vi "Read Config.vi"(10 "Config Path":path) -> (0 "Test Table":string[][](array[string]), 1 "C_Tol":dbl, 2 "P_Tol":dbl, 3 "PSID":dbl, 5 "Excel  Template":path)   [LabVIEW 2018]
uses:
  <vilib>/Utility/config.llb/Read Key (Double).vi
  <vilib>/Utility/config.llb/Read Key (Path).vi
  <vilib>/Utility/config.llb/Read Key (String).vi
  <vilib>/Utility/config.llb/NI_LVConfig.lvlib
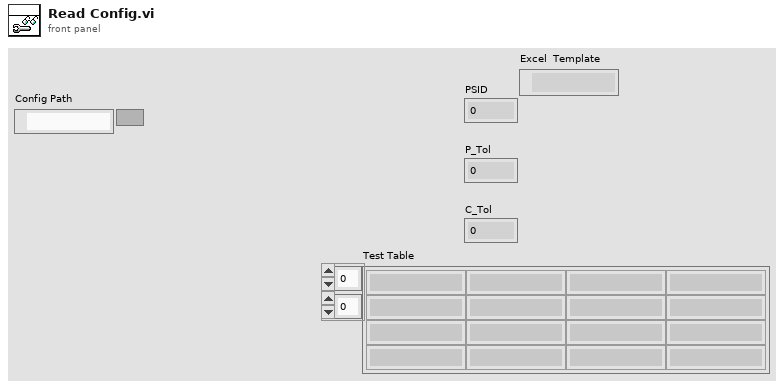
[diagram p1: front panel]
types:
  T1 = typedef "NI_LVConfig.lvlib/Config Data RefNum.ctl" = refnum<k1>
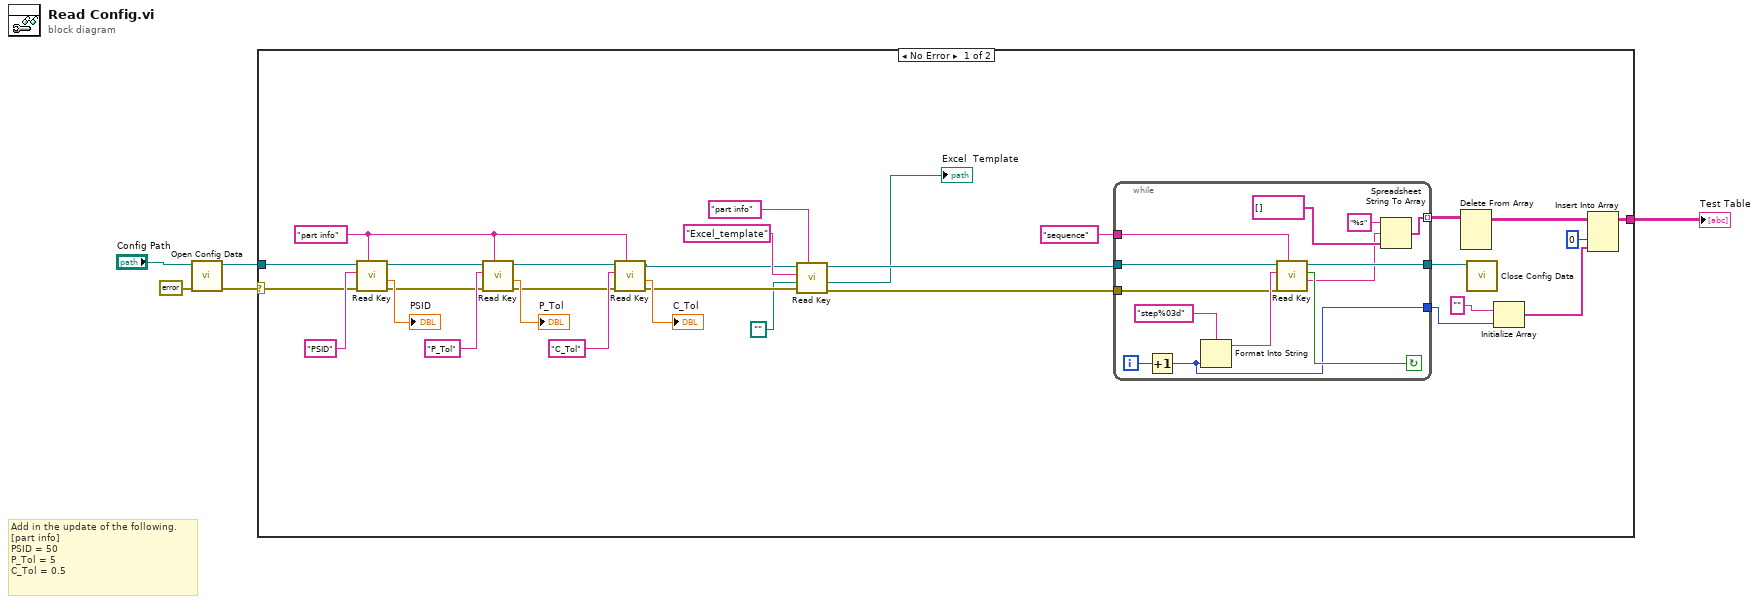
[diagram p0: block diagram]
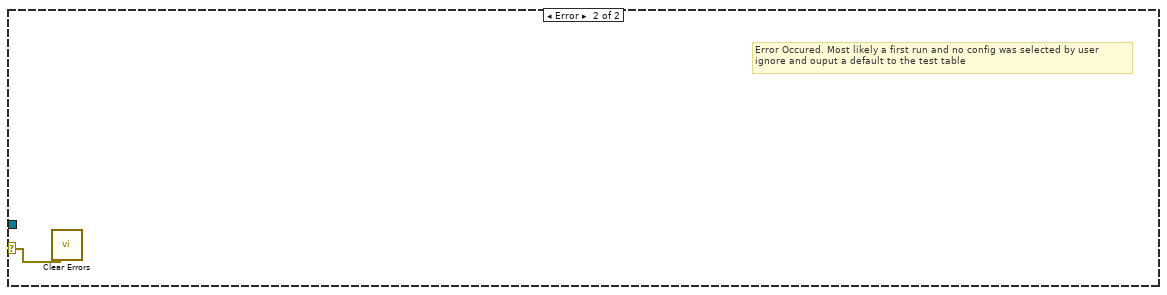
[diagram p2: hidden frame]
diagram:
  # "Add in the update of the following.\n[part info]\nPSID = 50\nP_Tol = 5\nC_Tol = 0.5"
  n1 = call <vilib>:"Open Config Data.vi"("error in (no error)"=errorcluster {"status"=FALSE, "code"=0, "source"=""}, "configuration file path"="Config Path") -> ("error out"=w2:errorcluster, "refnum"=w5:T1)  [unwired: 7 in, 1 out]
  n2 = case shown="No Error" w2 {
    selector: w2 -> [w13 w49]
    tunnel: w5 -> [w35 _]
    tunnel: [w21 _] -> w4
    frame No Error {
      w34 = "part info" ("section")
      n3 = call-poly <vilib>:"Read Key.vi"("section"=w34, "error in (no error)"=w13, "key"="PSID", "refnum"=w35) -> ("error out"=w12:errorcluster, "value"=→"PSID":dbl, "refnum out"=w27:T1)  [unwired: 4 in, 1 out]
      n4 = call-poly <vilib>:"Read Key.vi"("section"=w34, "error in (no error)"=w12, "key"="P_Tol", "refnum"=w27) -> ("error out"=w11:errorcluster, "value"=→"P_Tol":dbl, "refnum out"=w26:T1)  [unwired: 4 in, 1 out]
      n5 = call-poly <vilib>:"Read Key.vi"("section"=w34, "error in (no error)"=w11, "key"="C_Tol", "refnum"=w26) -> ("error out"=w10:errorcluster, "value"=→"C_Tol":dbl, "refnum out"=w14:T1)  [unwired: 4 in, 1 out]
      n6 = call-poly <vilib>:"Read Key.vi"("section"="part info", "error in (no error)"=w10, "default value"=path "", "key"="Excel_template", "refnum"=w14) -> ("error out"=w9:errorcluster, "value"=→"Excel  Template":path, "refnum out"=w8:T1)  [unwired: 3 in, 1 out]
      n7 = while {
        tunnel: w8 -> [w48]
        tunnel: "sequence" ("section") -> [w47]
        tunnel: [w42] -> w24
        tunnel: [w39] -> w23 mode=indexing
        tunnel: [w37] -> w20
        tunnel: w9 -> [w36]
        i -> [w46]
        stop <- w43 continue-if-true
        n8 = Increment(x=w46) -> (x+1=w37:i32)
        n9 = Format Into String(format string="step%03d", w37) -> (resulting string=w44:string)  [unwired: 2 in, 1 out]
        n10 = call-poly <vilib>:"Read Key.vi"("section"=w47, "error in (no error)"=w36, "key"=w44, "refnum"=w48) -> ("value"=w40:string, "found?"=w43:bool, "refnum out"=w42:T1)  [unwired: 4 in, 1 out]
        n11 = Spreadsheet String To Array(format string="%s", spreadsheet string=w40, array type (2D Dbl)=string[] []) -> (array=w39:string[])  [unwired: 1 in]
      }
      n12 = Delete From Array(array=w23) -> (array with subset deleted=w22:string[][])  [unwired: 3 in, 1 out]
      n13 = call <vilib>:"Close Config Data.vi"("refnum"=w24) -> ()  [unwired: 9 in, 2 out]
      n14 = Initialize Array("", w20) -> (w18:string[])
      n15 = Insert Into Array(array=w22, index (col)=0 ("disabled index (col)"), new element=w18) -> (w21:string[][])  [unwired: 1 in]
    }
    frame Error {
      # "Error Occured. Most likely a first run and no config was selected by user\nignore and ouput a default to the test table"
      n16 = call <vilib>:"Clear Errors.vi"("error in (no error)"=w49) -> ()  [unwired: 5 in, 2 out]
    }
  }
  "Test Table" <- w4
